vi "BuildMsgAnalogReporting.vi"(8 "error in":errorcluster, 9 "Enable Reporting?":bool, 10 "Pin Index":u8 format="%x") -> (0 "error out":errorcluster, 1 "ReplyLength":i32=-1, 2 "ReplyFirstByte":T1=224 items=["ANALOG_IO_MESSAGE"=224, "DIGITAL_IO_MESSAGE"=144, "REPORT_ANALOG_PIN"=192, "REPORT_DIGITAL_PORT"=208, "START_SYSEX"=240, "END_SYSEX"=247, "SET_PIN_MODE"=244, "SET_DIGITAL_PIN_VALUE"=245, "PROTOCOL_VERSION"=249, "SYSTEM_RESET"=255, "SYSEX.EXTENDED_ID"=0, "SYSEX.RESERVED_USER_COMMANDs"=1, "SYSEX.ANALOG_MAPPING_QUERY"=105, "SYSEX.ANALOG_MAPPING_RESPONSE"=106, "SYSEX.CAPABILITY_QUERY"=107, "SYSEX.CAPABILITY_RESPONSE"=108, "SYSEX.PIN_STATE_QUERY"=109, "SYSEX.PIN_STATE_RESPONSE"=110, "SYSEX.REPORT_FIRMWARE"=121, "SYSEX.EXTENDED_ANALOG"=111, "SYSEX.STRING_DATA"=113, "SYSEX.REALTIME"=127, "SYSEX.NON_REALTIME"=126, "SYSEX.SAMPLING_INTERVAL"=122], 3 "AnalogReportingMessage":u8[](array[numeric]) format="%x")   [LabVIEW 2020, in "FirmataClient.lvlib"]
doc: "Builds the message according to the Firmata Protocol Requirements. \n- https://github.com/firmata/protocol\n- https://github.com/firmata/protocol/blob/master/protocol.md"
uses:
  FirmataClient.lvlib
  controls/FirmataProtocolConstants.ctl
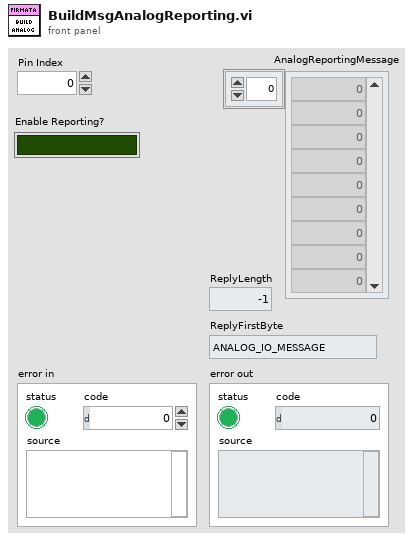
[diagram p1: front panel]
types:
  T1 = typedef "FirmataClient.lvlib/FirmataProtocolConstants.ctl" = u16
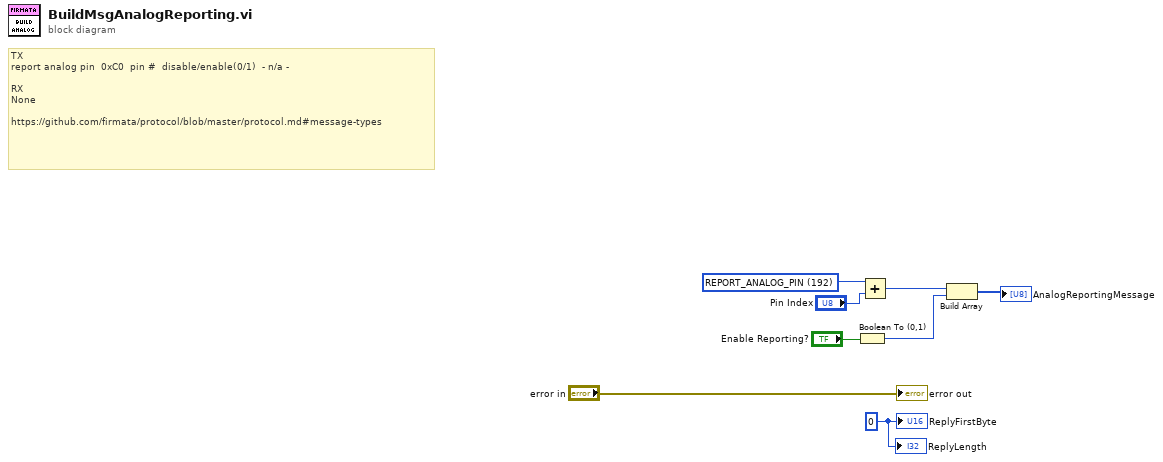
[diagram p0: block diagram]
diagram:
  w1 = 0
  w2 = T1 192 items=["ANALOG_IO_MESSAGE"=224, "DIGITAL_IO_MESSAGE"=144, "REPORT_ANALOG_PIN"=192, "REPORT_DIGITAL_PORT"=208, "START_SYSEX"=240, "END_SYSEX"=247, "SET_PIN_MODE"=244, "SET_DIGITAL_PIN_VALUE"=245, "PROTOCOL_VERSION"=249, "SYSTEM_RESET"=255, "SYSEX.EXTENDED_ID"=0, "SYSEX.RESERVED_USER_COMMANDs"=1, "SYSEX.ANALOG_MAPPING_QUERY"=105, "SYSEX.ANALOG_MAPPING_RESPONSE"=106, "SYSEX.CAPABILITY_QUERY"=107, "SYSEX.CAPABILITY_RESPONSE"=108, "SYSEX.PIN_STATE_QUERY"=109, "SYSEX.PIN_STATE_RESPONSE"=110, "SYSEX.REPORT_FIRMWARE"=121, "SYSEX.EXTENDED_ANALOG"=111, "SYSEX.STRING_DATA"=113, "SYSEX.REALTIME"=127, "SYSEX.NON_REALTIME"=126, "SYSEX.SAMPLING_INTERVAL"=122] ("FimataProtocolConstants")
  # "TX\nreport analog pin \t0xC0 \tpin # \tdisable/enable(0/1) \t- n/a -\n\nRX\nNone\n\nhttps://github.com/firmata/protocol/blob/master/protocol.md#message-types"
  n1 = Boolean To (0,1)(Boolean="Enable Reporting?") -> (0, 1=w3:i16)
  n2 = Add(x=w2, y="Pin Index") -> (x+y=w6:T1)
  n3 = Build Array(w6, w3) -> (→"AnalogReportingMessage":T1[])
  "error out" <- "error in"
  "ReplyFirstByte" <- w1
  "ReplyLength" <- w1
